vi "Write stopMessage.vi"(8 "error in (no error)":errorcluster, 10 "stopMessage":string="stop", 11 "MsgUETaskChannel in":refnum<class "MsgUETaskChannel.lvclass">) -> (0 "error out":errorcluster, 3 "MsgUETaskChannel out":refnum<class "MsgUETaskChannel.lvclass">)   [LabVIEW 2023, in "TLC_Daemon.lvlib" / "MsgUETaskChannel.lvclass"]
uses:
  MsgUETaskChannel.lvclass
  MsgUETaskChannel.lvclass/MsgUETaskChannel.ctl
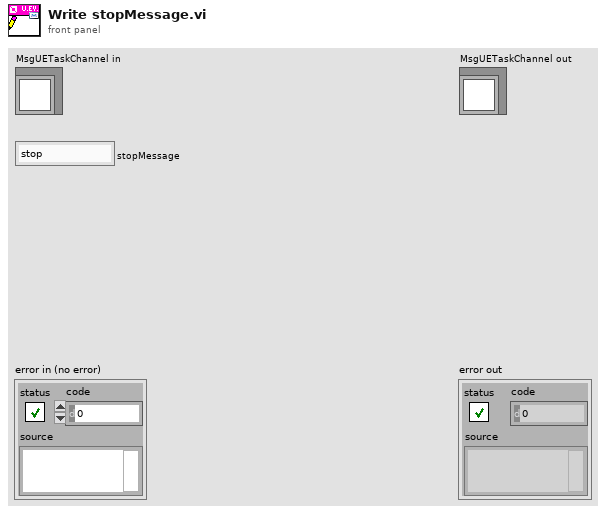
[diagram p1: front panel]
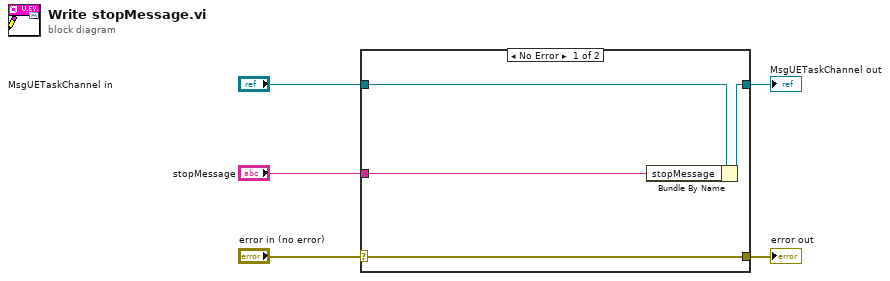
[diagram p0: block diagram]
diagram:
  n1 = case shown="No Error" "error in (no error)" {
    selector: "error in (no error)" -> [w9 w10]
    tunnel: [w9 w10] -> w4
    tunnel: [w7 w11] -> w2
    tunnel: "MsgUETaskChannel in" -> [w8 w11]
    tunnel: "stopMessage" -> [w6 _]
    frame No Error {
      n2 = Bundle By Name(cluster=w8, "stopMessage"=w6) -> (w7:refnum<class "MsgUETaskChannel.lvclass">)
    }
    frame Error {
    }
  }
  "error out" <- w4
  "MsgUETaskChannel out" <- w2
